vi "GetConfigChain.vi"(8 "error in (no error)":errorcluster, 11 "reference in":refnum<class "DMM_Keysight_34980A.lvclass">) -> (0 "error out":errorcluster, 2 "Config out":string[](array[string]), 3 "reference out":refnum<class "DMM_Keysight_34980A.lvclass">)   [LabVIEW 2022 SP3, in "DMM_Keysight_34980A.lvlib" / "DMM_Keysight_34980A.lvclass"]
uses:
  DMM_Keysight_34980A.lvclass
  Components/ViPER.lvlibp/ViPER.lvclass
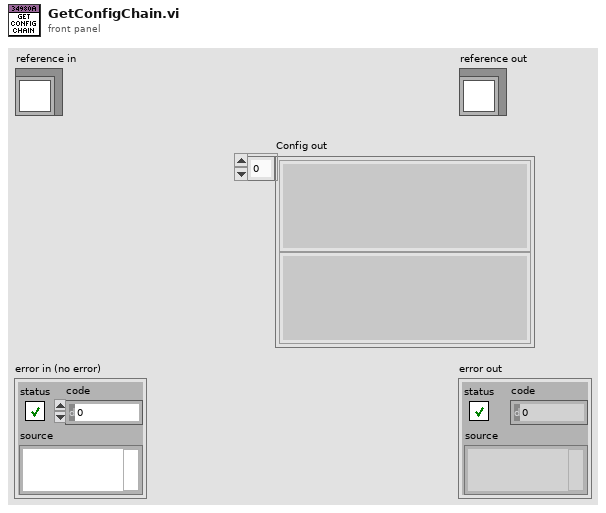
[diagram p1: front panel]
types:
  T1 = typedef "DMM_Keysight_34980A.lvlib/DMM_Keysight_34980A.lvclass/ObjectAttributes.ctl" = cluster{"Config":T2, "VISA ref":refnum<visa-resource-name>, "Meas":dbl, "Range DCV":enum16{"100 mV", "1 V", "10 V", "100 V", "300 V", "Auto", "Minimum", "Maximum"}, "Range ACV":enum16{"100 mV", "1 V", "10 V", "100 V", "300 V", "Auto", "Minimum", "Maximum", "Default"}, "Range Ohms":enum16{"100 Ohm", "1 kOhm", "10 kOhm", "100 kOhm", "1 MOhm", "10 MOhm", "100 MOhm", "Auto", "Minimum", "Maximum"}, "Range VFreq":enum16{"100 mV", "1 V", "10 V", "100 V", "300 V", "Auto", "Minimum", "Maximum"}, " Range ACA":enum16{"10 mA", "100 mA", "1 A", "Auto", "Minimum", "Maximum"}, " Range DCA":enum16{"10 mA", "100 mA", "1 A", "Auto", "Minimum", "Maximum"}, "Mode":T3, "Resolution":enum16{"4 1/2", "5 1/2", "6 1/2", "Least", "Highest", "Default"}, "Bandwidth":enum16{"3 Hz", "20 Hz", "200 Hz", "Minimum", "Maximum"}, "Low Frequency":enum16{"3 Hz", "20 Hz", "200 Hz", "Minimum", "Maximum"}, "Aperture":enum16{"10 ms", "100 ms", "1 sec", "Minimum", "Maximum"}, "Measurement":dbl[], "Time":dbl[], "Samples":u32, "dt":dbl, "Timeout":dbl}
  T2 = typedef "DMM_Keysight_34980A.lvlib/DMM_Keysight_34980A.lvclass/Config.ctl" = cluster{"VISA":refnum<visa-resource-name>}
  T3 = typedef "DMM_Keysight_34980A.lvlib/DMM_Keysight_34980A.lvclass/Mode.ctl" = enum16{"DCV", "ACV", "2W Ohms", "4W Ohms", "Frequency", "DCA", "ACA"}
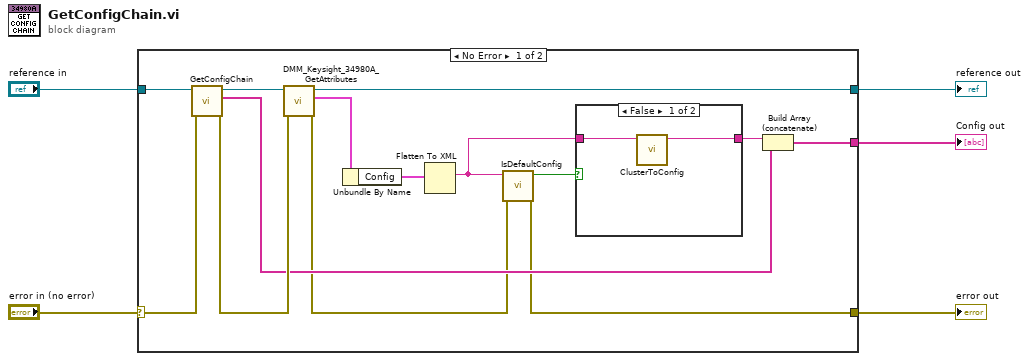
[diagram p0: block diagram]
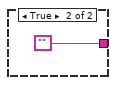
[diagram p2: hidden frame]
diagram:
  n1 = case shown="No Error" "error in (no error)" {
    selector: "error in (no error)" -> [w15 w24]
    tunnel: [w6 w24] -> w4
    tunnel: [w13 w23] -> w2
    tunnel: "reference in" -> [w17 w23]
    tunnel: [w10 _] -> w1
    frame No Error {
      n2 = call-parent "GetConfigChain.vi"("error in (no error)"=w15, "reference in"=w17) -> ("error out"=w14:errorcluster, "Config out"=w11:string[], "reference out"=w16:refnum<class "DMM_Keysight_34980A.lvclass">)  [unwired: 7 in]
      n3 = call "DMM_Keysight_34980A_GetAttributes.vi"("error in (no error)"=w14, "reference in"=w16) -> ("error out"=w7:errorcluster, "Data"=w19:T1, "reference out"=w13:refnum<class "DMM_Keysight_34980A.lvclass">)  [unwired: 6 in, 1 out]
      n4 = Unbundle By Name(w19) -> ("Config"=w18:T2)
      n5 = Flatten To XML(6:w18) -> (2:w9:string)
      n6 = call "IsDefaultConfig.vi"("error in (no error)"=w7, "Config XML"=w9) -> ("error out"=w6:errorcluster, "Is Default"=w8:bool)  [unwired: 8 in]
      n7 = case shown="False" w8 {
        tunnel: w9 -> [w21 _]
        tunnel: [w20 ""] -> w12
        frame False {
          n8 = call "ClusterToConfig.vi"("Cluster XML"=w21) -> ("Config XML"=w20:string)  [unwired: 10 in]
        }
        frame True {
        }
      }
      n9 = Build Array (concatenate)(w12, w11) -> (w10:string[])
    }
    frame Error {
    }
  }
  "error out" <- w4
  "reference out" <- w2
  "Config out" <- w1
